vi "GetFrameworkDefaultSubpanelPath.vi"(8 "error in (no error)":errorcluster, 11 "SMO.UI.MAUI in":refnum<class "SMO.UI.MAUI.lvclass">) -> (0 "error out":errorcluster, 2 "path":path, 3 "SMO.UI.MAUI out":refnum<class "SMO.UI.MAUI.lvclass">)   [LabVIEW 2019, in "SMO.UI.MAUI.lvclass"]
doc: "Will get the path of the subpanel that the framework uses as a default. This reads from the default configuration file. If it is not found, then it will generate a path based on a constant location."
uses:
  SMO.UI.MAUI.lvclass
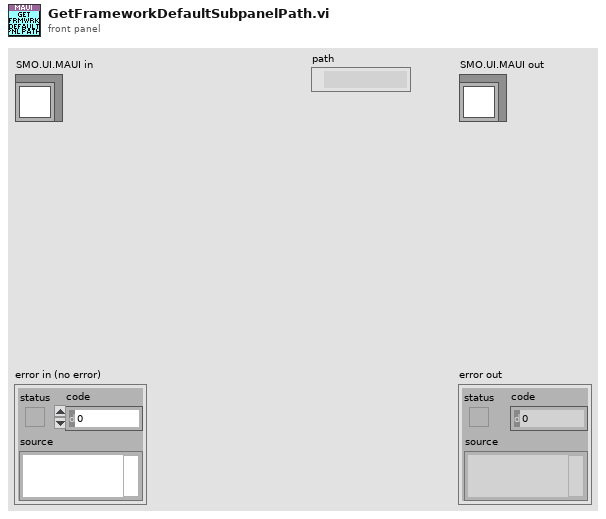
[diagram p1: front panel]
types:
  T1 = typedef "SMO.UI.MAUI.lvclass/DefaultConfiguration.ctl" = cluster{"Default Subpanel":string}
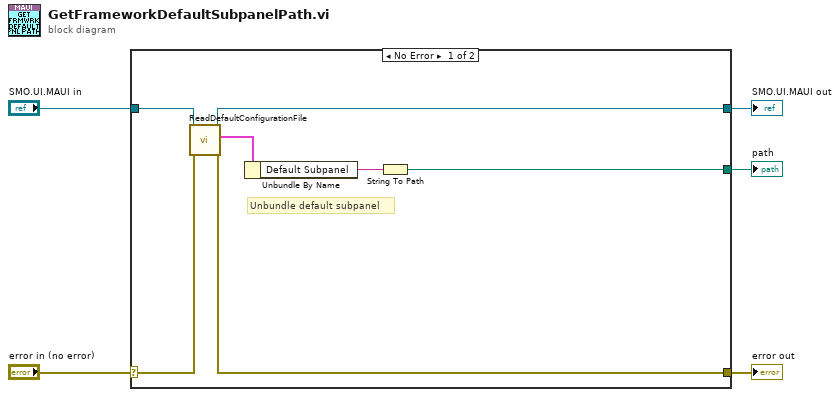
[diagram p0: block diagram]
diagram:
  n1 = case shown="No Error" "error in (no error)" {
    selector: "error in (no error)" -> [w10 w14]
    tunnel: [w9 w14] -> w4
    tunnel: [w12 w13] -> w2
    tunnel: "SMO.UI.MAUI in" -> [w11 w13]
    tunnel: [w6 _] -> w1
    frame No Error {
      # "Unbundle default subpanel"
      n2 = call "ReadDefaultConfigurationFile.vi"("error in (no error)"=w10, "SMO.UI.MAUI in"=w11) -> ("error out"=w9:errorcluster, "Default Data"=w8:T1, "SMO.UI.MAUI out"=w12:refnum<class "SMO.UI.MAUI.lvclass">)  [unwired: 7 in]
      n3 = Unbundle By Name(w8) -> ("Default Subpanel"=w7:string)
      n4 = String To Path(string=w7) -> (path=w6:path)
    }
    frame Error {
    }
  }
  "error out" <- w4
  "SMO.UI.MAUI out" <- w2
  "path" <- w1
